vi "Gestion Shielding Box.vi"() -> ()   [LabVIEW 2020]
uses:
  Commun VI/TypeDef/Commande Popup autotest/Commande element autotest.ctl
  <vilib>/Instr/_visa.llb/Select Event Type.ctl
  <vilib>/Instr/_visa.llb/VISA Event Mechanism.ctl
  Action.ctl
  Commande special/Exit.ctl
  IHM/Variable globale.vi
panel:
  out "Element autotest":T1
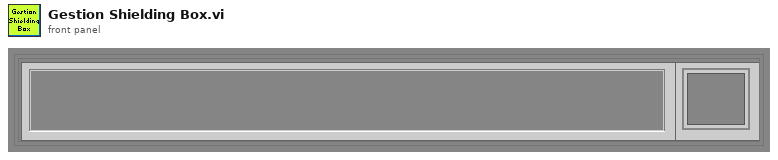
[diagram p1: front panel]
types:
  T1 = typedef "Commande element autotest.ctl" = cluster{"Instrument":string, "Etat":cluster{"Menu déroulant":u16}}
  T2 = typedef "Action.ctl" = enum16{"Open Shielding", "Close Shielding", "Read Status", "Stop Wait Start", "Wait Start", "Wait Close", "Wait Open", "Quit"}
  T3 = typedef "File et notification.ctl" = cluster{"Arret Appli":refnum<notifier>, "Erreur Acqui":refnum<notifier>, "File Event Sequenceur":refnum<queue>, "Liste test à faire":refnum<queue>, "File Event Historique":refnum<queue>, "Variable Global":refnum<notifier>, "Variable stocke retour Etat":refnum<notifier>, "Retour Validation OP":refnum<queue>, "Demande Validation OP":refnum<queue>, "Retour Autotest":refnum<notifier>, "Demande Autotest":refnum<queue>, "Adr Mac Produit":refnum<notifier>, "Autorise commande":refnum<notifier>, "Event Init BLE":refnum<notifier>, "Action Lecture RS":refnum<queue>, "Key produit":refnum<notifier>, "Retour Saisie OP":refnum<queue>, "Demande Saisie OP":refnum<queue>, "Etat flashage":refnum<notifier>, "Code Operateur":refnum<notifier>, "Resultat test Global":refnum<notifier>, "Stop Test":refnum<notifier>, "Init IHM Autotest":refnum<notifier>, "Version test bench":refnum<notifier>, "SN Product":refnum<notifier>, "En erreur":refnum<notifier>, "Affiche Result":refnum<queue>, "S/N PWR":refnum<notifier>, "AppEUI":refnum<notifier>, "Action Lecture Temp":refnum<queue>, "Temp":refnum<notifier>, "AppKey":refnum<notifier>, "OF":refnum<notifier>, "File Commande Shielding":refnum<queue>, "Return Status":refnum<notifier>, "ID Product":refnum<notifier>, "Version FW":refnum<notifier>, "Version HW":refnum<notifier>, "Adresse IHM":refnum<notifier>, "RTC":refnum<notifier>, "S/N Ant":refnum<notifier>, "SN Encode":refnum<notifier>, "Key Product":refnum<notifier>}
  T4 = typedef "Commande Variable Global.ctl" = cluster{"Fichier":cluster{"Chemin Save Historique":path, "Fichier Appplication":string, "Fichier Test":string, "Fichier Langue":string, "Part Number":string, "Fichier Parametre":string, "Chemin Fichier Parametre":path, "Fichier Print":string, "Fichier BDD":string}, "Liaison Serie":cluster{"RS Alimentation":refnum<visa-resource-name>, "RS Multimetre":refnum<k15>, "RS Carte":refnum<visa-resource-name>, "RS Dongle WIFI":refnum<visa-resource-name>, "RS Dongle BLE":refnum<visa-resource-name>, "RSA306":refnum<visa-resource-name>, "RS Printer PCBA":refnum<visa-resource-name>, "RS Golden Sample":refnum<visa-resource-name>, "RS Printer Ass":refnum<visa-resource-name>, "RS Printer Pack":refnum<visa-resource-name>, "RS Sonde Temp":refnum<visa-resource-name>, "RS Multimetre Bis":refnum<k15>, "RS FEASA LED":refnum<visa-resource-name>}, "Liaison DIO":cluster{"Jlink":cluster{"Line":tag, "Nom Voie":string, "Nom device in INI":string}[], "ICD":cluster{"Line":tag, "Nom Voie":string, "Nom device in INI":string}[], "UART":cluster{"Line":tag, "Nom Voie":string, "Nom device in INI":string}[], "Multi1":cluster{"Line":tag, "Nom Voie":string, "Nom device in INI":string}[], "Multi2":cluster{"Line":tag, "Nom Voie":string, "Nom device in INI":string}[], "Multi3":cluster{"Line":tag, "Nom Voie":string, "Nom device in INI":string}[], "DO1":cluster{"Line":tag, "Nom Voie":string, "Nom device in INI":string}[], "DO2":cluster{"Line":tag, "Nom Voie":string, "Nom device in INI":string}[], "DO3":cluster{"Line":tag, "Nom Voie":string, "Nom device in INI":string}[], "AlimProduct":cluster{"Line":tag, "Nom Voie":string, "Nom device in INI":string}[], "SW2":cluster{"Line":tag, "Nom Voie":string, "Nom device in INI":string}[], "SW1":cluster{"Line":tag, "Nom Voie":string, "Nom device in INI":string}[], "Multi220V_CPT":cluster{"Line":tag, "Nom Voie":string, "Nom device in INI":string}[]}, "Variable Programme":T5, "Information Entete":cluster{"Opérateur":string, "Ordre de fabrication":string, "Numéro de lot":string, "Commentaire":string}, "Nom de périphérique DAQmx":tag, "Parameter RF":cluster{"Frequency CW":string, "FrequencyRX":string, "TimeOutRX":string}, "Divers":cluster{"DUT Hub":u32}, "Analogique":cluster{"AI1":cluster{"Voie":tag, "Nom Voie":string, "Nom device in INI":string}[], "Ai2":cluster{"Voie":tag, "Nom Voie":string, "Nom device in INI":string}[], "AI3":cluster{"Voie":tag, "Nom Voie":string, "Nom device in INI":string}[], "AI4":cluster{"Voie":tag, "Nom Voie":string, "Nom device in INI":string}[], "AI5":cluster{"Voie":tag, "Nom Voie":string, "Nom device in INI":string}[], "AI6":cluster{"Voie":tag, "Nom Voie":string, "Nom device in INI":string}[], "AI7":cluster{"Voie":tag, "Nom Voie":string, "Nom device in INI":string}[], "AI8":cluster{"Voie":tag, "Nom Voie":string, "Nom device in INI":string}[], "AO1":cluster{"Voie":tag, "Nom Voie":string, "Nom device in INI":string}[], "AO2":cluster{"Voie":tag, "Nom Voie":string, "Nom device in INI":string}[]}, "Parametre BLE":T8, "Shielding Box":cluster{"Comm":refnum<visa-resource-name>, "Used":bool}, "Challenge Bit":u8[]}
  T5 = typedef "Commande Variables Programme.ctl" = cluster{"Cigarette en cours":i32, "Tableau Resultat test":T6, "Test en cours":i32, "Type test":string, "Type Carte":T7, "Test Select":cluster{"Booléen 4":bool}[]}
  T6 = typedef "Commande tableau Resultat.ctl" = cluster{"Resultat produit":cluster{"Nom test":string, "Result test":bool[], "Nom pointe de test":string[], "Valeur test":string[], "Temps Etape":dbl, "Numero Etape":string[]}[]}[]
  T7 = typedef "Commande Selection produit en cours.ctl" = enum16{"None", "PCBA", "Assembled"}
  T8 = typedef "Comande Variable Globale BLE.ctl" = cluster{"Devices Connect":string[][], "Connection Status":T9, "Handle table":string[][], "Service":string, "characteristic Read":string, "characteristic Write":string, "Port BLE":refnum<visa-resource-name>, "Nb Packet Light":u8}
  T9 = typedef "connection_status_bundle.ctl" = cluster{"MAC Address":string, "cnx handle":u8, "cnx flags":u8, "Address Type":T10, "Connection Interval (ms)":u16, "Timeout(ms)":u16, "Latency":u16, "bonding handle":u8}
  T10 = typedef "address_type.ctl" = u8
  T11 = typedef "Exit.ctl" = bool
  T12 = enum32{"Invalid", "Standard", "Closed", "Hidden", "Minimized", "Maximized"}
  T13 = typedef "VISA Event Mechanism.ctl" = u16
  T14 = typedef "Select Event Type.ctl" = u32
  T15 = typedef "Adresse IHM.ctl" = cluster{"TabGestionScénario":refnum<vi>, "MAJ TabTest":refnum<vi>, "MAJ IHM":refnum<vi>, "BpStop":refnum<vi>, "Autotest OK":refnum<vi>, "BpContinue":refnum<vi>, "BpStart":refnum<vi>, "Action en chinois":refnum<vi>, "Bouton vide":refnum<vi>, "StatusPCB":refnum<vi>, "StatusAssembled":refnum<vi>, "Bouton Exit":refnum<vi>, "Action En cours":refnum<vi>}
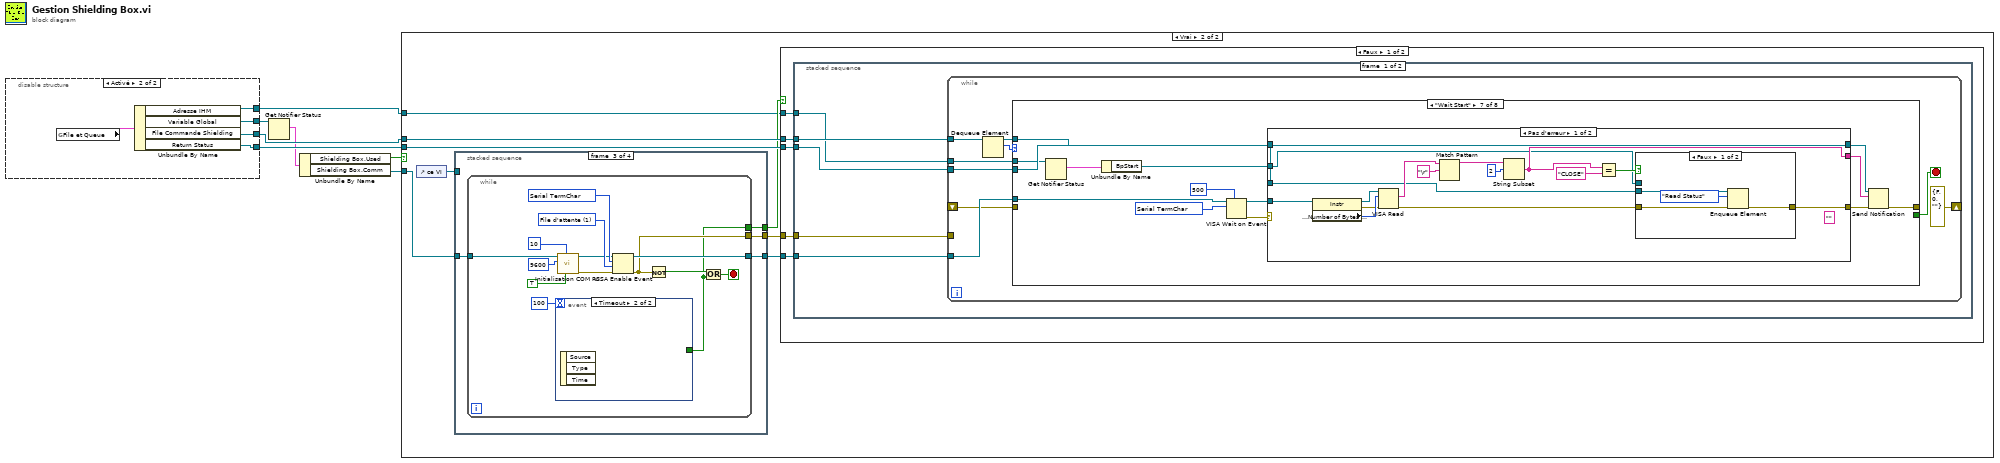
[diagram p0: block diagram]
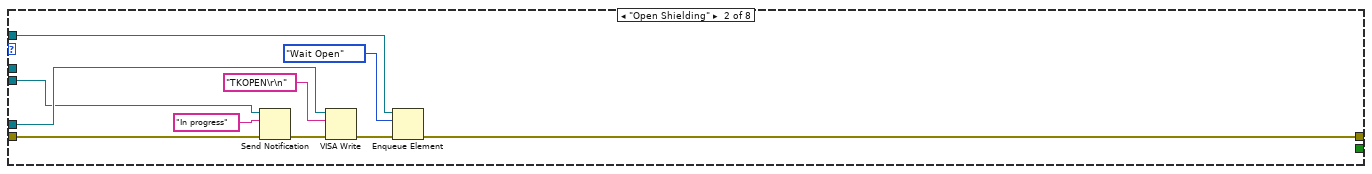
[diagram p4: hidden frame]
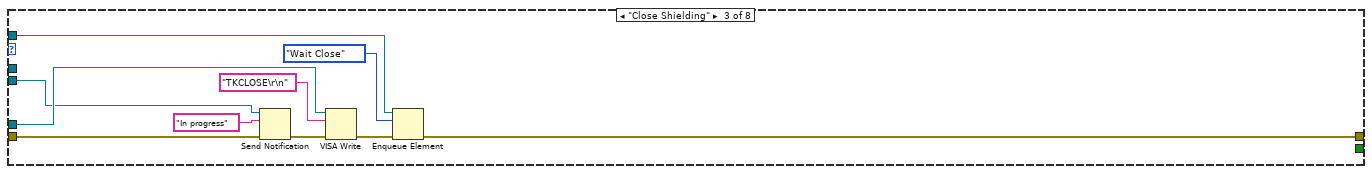
[diagram p5: hidden frame]
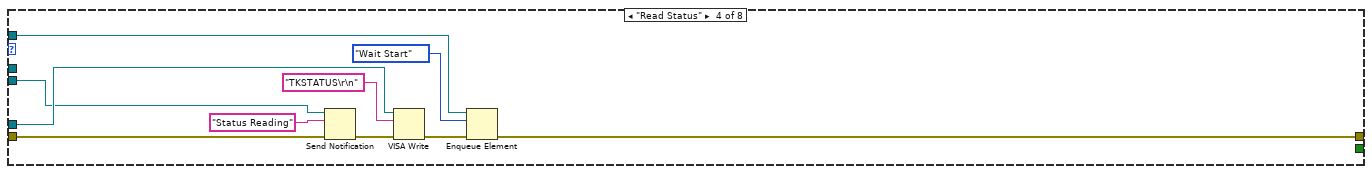
[diagram p6: hidden frame]
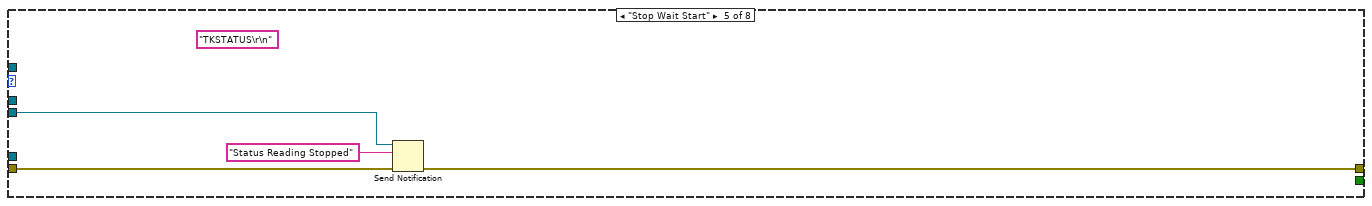
[diagram p7: hidden frame]
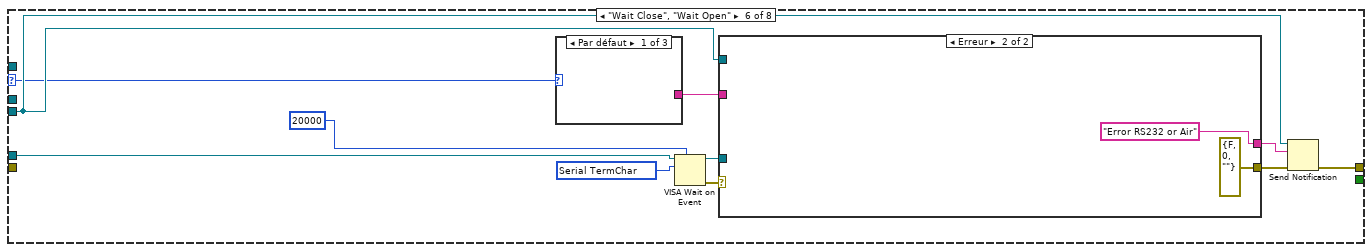
[diagram p8: hidden frame]
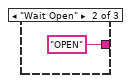
[diagram p9: hidden frame]
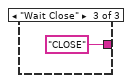
[diagram p10: hidden frame]
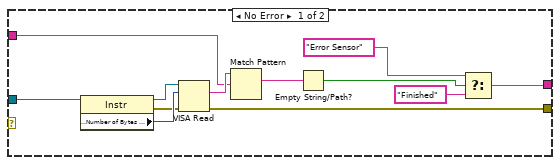
[diagram p11: hidden frame]
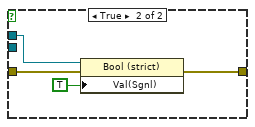
[diagram p12: hidden frame]
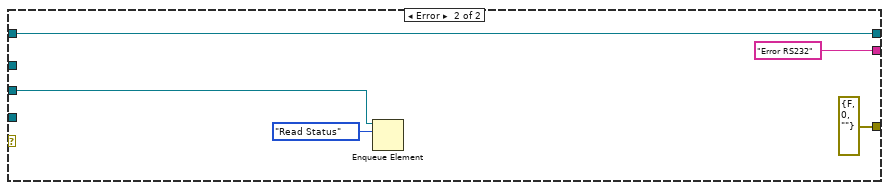
[diagram p13: hidden frame]
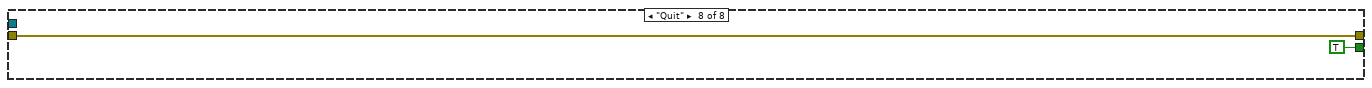
[diagram p14: hidden frame]
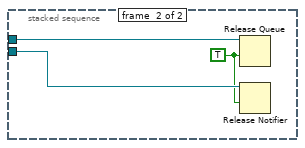
[diagram p15: hidden frame]
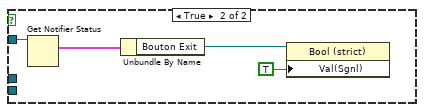
[diagram p16: hidden frame]
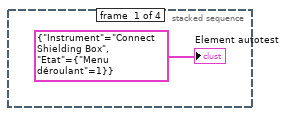
[diagram p17: hidden frame]
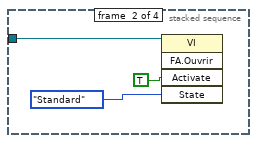
[diagram p18: hidden frame]
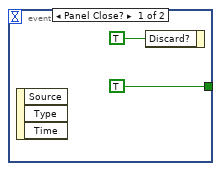
[diagram p19: hidden frame]
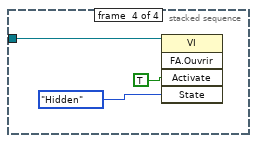
[diagram p20: hidden frame]
diagram:
  n1 = disable-structure shown="Activé" {
    disable-tunnel: [w12 w17] -> w7
    disable-tunnel: [w9 w16] -> w6
    disable-tunnel: [_ w15] -> w5
    disable-tunnel: [_ w14] -> w1
    frame Disabled {
      n2 = Obtain Queue(name (unnamed)="File Commande Shielding" ("nom (aucun)"), element data type=Action."Wait Start") -> (queue out=w12:refnum<queue>)  [unwired: 3 in, 2 out]
      n3 = Obtain Notifier(name (unnamed)="Return Status" ("nom (aucun)"), notification data type="") -> (notifier out=w9:refnum<notifier>)  [unwired: 2 in, 2 out]
    }
    frame Enabled {
      n4 = global read "Variable globale.vi" "File et Queue"() -> (w18:T3)
      n5 = Unbundle By Name(w18) -> ("Adresse IHM"=w14:refnum<notifier>, "Variable Global"=w15:refnum<notifier>, "File Commande Shielding"=w17:refnum<queue>, "Return Status"=w16:refnum<notifier>)
    }
  }
  n6 = Get Notifier Status(notifier=w5) -> (current notification=w3:T4)  [unwired: 1 in, 4 out]
  n7 = Unbundle By Name(w3) -> ("Shielding Box.Used"=w2:bool, "Shielding Box.Comm"=w4:refnum<visa-resource-name>)
  n8 = case shown="Vrai" w2 {
    tunnel: w7 -> [_ w26]
    tunnel: w6 -> [_ w25]
    tunnel: w1 -> [_ w20]
    tunnel: w4 -> [_ w19]
    frame False {
    }
    frame True {
      n9 = control-ref of="ce VI"() -> (w24:refnum<vi>)
      n10 = stacked-sequence {
        tunnel: w24 -> [_ w161 _ w184]
        tunnel: [_ _ w167 _] -> w23
        tunnel: [_ _ w166 _] -> w22
        tunnel: [_ _ w165 _] -> w21
        tunnel: w19 -> [_ _ w164 _]
        frame #0 {
          "Element autotest" <- T1 {"Instrument"="Connect Shielding Box", "Etat"={"Menu déroulant"=1}} ("Element autotest")
        }
        frame #1 {
          n11 = invoke class="VI" method="FA.Ouvrir"(reference=w161, "Activate"=TRUE ("Activer ?"), "State"=T12."Standard" ("État")) -> ()  [unwired: 2 in, 5 out]
        }
        frame #2 {
          n12 = while {
            tunnel: [w172] -> w167
            tunnel: [w174] -> w166
            tunnel: [w170] -> w165
            tunnel: w164 -> [w168]
            stop <- w173 stop-if-true
            w177 = T13 1 items=["File d'attente"=1] ("Mechanism Type")
            w176 = T14 1073684516 items=["Service Request"=1073684491, "Trigger"=3221168138, "Clear"=1073684493, "VXI Signal"=1073684512, "VXI/VME Interrupt"=3221168161, "VXI/VME Sysfail"=1073684509, "VXI/VME Sysreset"=1073684510, "GPIB-CIC"=1073684498, "GPIB-Talk"=1073684499, "GPIB-Listen"=1073684500, "PXI Interrupt"=1073684514, "Serial Break"=1073684515, "Serial TermChar"=1073684516, "Serial CTS"=1073684521, "Serial DSR"=1073684522, "Serial DCD"=1073684524, "Serial RI"=1073684526, "Serial Character"=1073684533, "USB Interrupt"=1073684535, "All Enabled"=1073709055] ("Event Type")
            n13 = event shown="[1] Timeout" {
              selector: _ -> [_ _]
              dyn-events: _ -> [_ _]
              timeout: 100 -> [_ _]
              tunnel: [TRUE _] -> w170
              event Panel Close? {
                n14 = event-data() -> ()  [unwired: 1 in, 3 out]
                n15 = event-data("Discard?"=TRUE ("Rejeter ?")) -> ()  [unwired: 1 in, 1 out]
              }
              event Timeout {
                n16 = event-data() -> ()  [unwired: 1 in, 3 out]
              }
            }
            n17 = call "Initialisation COM RS.vi"("Enable Termination\nChar (T)"=TRUE ("Enable Termination\nChar (T)"), "termination char\n(0xA = '\\n' = LF)"=u8 10 ("termination char\n(0xA = '\\n' = LF)"), "baud rate (9600)"=9600, "Refnum VISA en entrée"=w168) -> ("sortie d'erreur"=w178:errorcluster, "Nom de ressource VISA en sortie"=w175:refnum<visa-resource-name>)  [unwired: 6 in]
            n18 = VISA Enable Event(8:w178, 9:w177, 10:w176, 11:w175) -> (0:w172:errorcluster, 3:w174:refnum<visa-resource-name>)
            n19 = Not(x=w172) -> (.not. x?=w171:bool)
            n20 = Or(x=w171, y=w170) -> (x .or. y?=w173:bool)
          }
        }
        frame #3 {
          n21 = invoke class="VI" method="FA.Ouvrir"(reference=w184, "Activate"=TRUE ("Activer ?"), "State"=T12."Hidden" ("État")) -> ()  [unwired: 2 in, 5 out]
        }
      }
      n22 = case shown="Faux" w21 {
        tunnel: w26 -> [w31 _]
        tunnel: w25 -> [w30 _]
        tunnel: w23 -> [w29 _]
        tunnel: w22 -> [w28 _]
        tunnel: w20 -> [w27 w159]
        frame False {
          n23 = stacked-sequence {
            tunnel: w28 -> [w36 _]
            tunnel: w31 -> [w35 w155]
            tunnel: w29 -> [w34 _]
            tunnel: w30 -> [w33 w154]
            tunnel: w27 -> [w32 _]
            frame #0 {
              n24 = while {
                tunnel: w36 -> [w43]
                tunnel: w35 -> [w45]
                shift-right: [errorcluster {"status"=FALSE, "code"=0, "source"=""} ("error out")] -> _
                shift-left: _ -> [w42]
                tunnel: w34 -> [_]
                tunnel: w33 -> [w39]
                tunnel: w32 -> [w37]
                stop <- w40 stop-if-true
                n25 = Dequeue Element(queue=w45) -> (queue out=w41:refnum<queue>, element=w44:T2)  [unwired: 2 in, 2 out]
                n26 = case shown="\"Wait Start\"" w44 {
                  selector: w44 -> [_ _ _ _ _ w86 _ _]
                  tunnel: w43 -> [_ w56 w66 w76 _ w91 w121 _]
                  tunnel: w42 -> [w46 w54 w58 w68 w78 _ _ w152]
                  tunnel: [w46 w52 w63 w73 w77 w82 w114 w152] -> _
                  tunnel: w41 -> [_ w51 w62 w72 _ _ w110 _]
                  tunnel: [_ _ _ _ _ _ _ TRUE] -> w40
                  tunnel: w39 -> [_ w48 w59 w69 w79 w88 w118 _]
                  tunnel: w37 -> [_ _ _ _ _ _ w115 _]
                  frame Default {
                  }
                  frame "Open Shielding" {
                    n27 = Send Notification(notification="In progress", notifier=w48, error in (no error)=w54) -> (error out=w49:errorcluster)  [unwired: 1 out]
                    n28 = VISA Write(VISA resource name=w56, write buffer="TKOPEN\r\n" ("buffer d'écriture"), error in (no error)=w49) -> (error out=w53:errorcluster)  [unwired: 2 out]
                    n29 = Enqueue Element(queue=w51, element=Action."Wait Open" ("élément"), error in (no error)=w53) -> (error out=w52:errorcluster)  [unwired: 1 in, 2 out]
                  }
                  frame "Close Shielding" {
                    n30 = Send Notification(notification="In progress", notifier=w59, error in (no error)=w58) -> (error out=w57:errorcluster)  [unwired: 1 out]
                    n31 = VISA Write(VISA resource name=w66, write buffer="TKCLOSE\r\n" ("buffer d'écriture"), error in (no error)=w57) -> (error out=w64:errorcluster)  [unwired: 2 out]
                    n32 = Enqueue Element(queue=w62, element=Action."Wait Close" ("élément"), error in (no error)=w64) -> (error out=w63:errorcluster)  [unwired: 1 in, 2 out]
                  }
                  frame "Read Status" {
                    n33 = Send Notification(notification="Status Reading", notifier=w69, error in (no error)=w68) -> (error out=w67:errorcluster)  [unwired: 1 out]
                    n34 = VISA Write(VISA resource name=w76, write buffer="TKSTATUS\r\n" ("buffer d'écriture"), error in (no error)=w67) -> (error out=w74:errorcluster)  [unwired: 2 out]
                    n35 = Enqueue Element(queue=w72, element=Action."Wait Start" ("élément"), error in (no error)=w74) -> (error out=w73:errorcluster)  [unwired: 1 in, 2 out]
                  }
                  frame "Stop Wait Start" {
                    (unwired) "TKSTATUS\r\n" ("buffer d'écriture")
                    n36 = Send Notification(notification="Status Reading Stopped", notifier=w79, error in (no error)=w78) -> (error out=w77:errorcluster)  [unwired: 1 out]
                  }
                  frame "Wait Close", "Wait Open" {
                    w90 = T14 1073684516 items=["Service Request"=1073684491, "Trigger"=3221168138, "Clear"=1073684493, "VXI Signal"=1073684512, "VXI/VME Interrupt"=3221168161, "VXI/VME Sysfail"=1073684509, "VXI/VME Sysreset"=1073684510, "GPIB-CIC"=1073684498, "GPIB-Talk"=1073684499, "GPIB-Listen"=1073684500, "PXI Interrupt"=1073684514, "Serial Break"=1073684515, "Serial TermChar"=1073684516, "Serial CTS"=1073684521, "Serial DSR"=1073684522, "Serial DCD"=1073684524, "Serial RI"=1073684526, "Serial Character"=1073684533, "USB Interrupt"=1073684535, "All Enabled"=1073709055] ("Event Type")
                    n37 = case shown="Par défaut" w86 {
                      tunnel: [_ "OPEN" ("expression régulière") "CLOSE" ("expression régulière")] -> w85
                      frame Default {
                      }
                      frame "Wait Open" {
                      }
                      frame "Wait Close" {
                      }
                    }
                    n38 = VISA Wait on Event(7:u32 20000 ("timeout (0)"), 10:w90, 11:w91) -> (0:w87:errorcluster, 3:w89:refnum<visa-resource-name>)  [unwired: 2 in, 2 out]
                    n39 = case shown="Erreur" w87 {
                      tunnel: w89 -> [w105 _]
                      tunnel: w88 -> [_ _]
                      tunnel: w85 -> [w96 _]
                      tunnel: [w95 "Error RS232 or Air" ("cas faux")] -> w84
                      tunnel: [w94 errorcluster {"status"=FALSE, "code"=0, "source"=""} ("error out")] -> w83
                      frame No Error {
                        n40 = property class="Instr"(reference=w105) -> (reference out=w104:refnum<visa-resource-name>, error out=w101:errorcluster, "Serial Settings:Number of Bytes at Serial Port"=w103:u32)  [unwired: 1 in]
                        n41 = VISA Read(VISA resource name=w104, byte count=w103, error in (no error)=w101) -> (read buffer=w100:string, error out=w94:errorcluster)  [unwired: 2 out]
                        n42 = Match Pattern(string=w100, regular expression=w96) -> (match substring=w102:string)  [unwired: 1 in, 3 out]
                        n43 = Empty String/Path?(string/path=w102) -> (empty?=w97:bool)
                        n44 = Select(t="Error Sensor" ("notification"), s=w97, f="Finished" ("cas faux")) -> (s? t:f=w95:string)
                      }
                      frame Error {
                      }
                    }
                    n45 = Send Notification(notification=w84, notifier=w88, error in (no error)=w83) -> (error out=w82:errorcluster)  [unwired: 1 out]
                  }
                  frame "Wait Start" {
                    w120 = T14 1073684516 items=["Service Request"=1073684491, "Trigger"=3221168138, "Clear"=1073684493, "VXI Signal"=1073684512, "VXI/VME Interrupt"=3221168161, "VXI/VME Sysfail"=1073684509, "VXI/VME Sysreset"=1073684510, "GPIB-CIC"=1073684498, "GPIB-Talk"=1073684499, "GPIB-Listen"=1073684500, "PXI Interrupt"=1073684514, "Serial Break"=1073684515, "Serial TermChar"=1073684516, "Serial CTS"=1073684521, "Serial DSR"=1073684522, "Serial DCD"=1073684524, "Serial RI"=1073684526, "Serial Character"=1073684533, "USB Interrupt"=1073684535, "All Enabled"=1073709055] ("Event Type")
                    n46 = Get Notifier Status(notifier=w115) -> (current notification=w116:T15)  [unwired: 1 in, 4 out]
                    n47 = Unbundle By Name(w116) -> ("BpStart"=w111:refnum<vi>)
                    n48 = VISA Wait on Event(7:u32 500 ("timeout (0)"), 10:w120, 11:w121) -> (0:w117:errorcluster, 3:w119:refnum<visa-resource-name>)  [unwired: 2 in, 2 out]
                    n49 = case shown="Pas d'erreur" w117 {
                      tunnel: w119 -> [w137 _]
                      tunnel: w118 -> [w128 w148]
                      tunnel: [w127 "Error RS232" ("cas faux")] -> w112
                      tunnel: [w122 errorcluster {"status"=FALSE, "code"=0, "source"=""} ("error out")] -> w109
                      tunnel: [w128 w148] -> w113
                      tunnel: w111 -> [w125 _]
                      tunnel: w110 -> [w123 w146]
                      frame No Error {
                        (unwired) "" ("sous-chaîne")
                        n50 = property class="Instr"(reference=w137) -> (reference out=w136:refnum<visa-resource-name>, error out=w134:errorcluster, "Serial Settings:Number of Bytes at Serial Port"=w135:u32)  [unwired: 1 in]
                        n51 = VISA Read(VISA resource name=w136, byte count=w135, error in (no error)=w134) -> (read buffer=w133:string, error out=w124:errorcluster)  [unwired: 2 out]
                        n52 = Match Pattern(string=w133, regular expression="\r" ("expression régulière")) -> (before substring=w131:string)  [unwired: 1 in, 3 out]
                        n53 = String Subset(string=w131, offset (0)=2) -> (substring=w127:string)  [unwired: 1 in]
                        n54 = Equal?(x=w127, y="CLOSE") -> (x = y?=w126:bool)
                        n55 = case shown="Faux" w126 {
                          tunnel: w125 -> [_ w145]
                          tunnel: w124 -> [w141 w143]
                          tunnel: [w140 w142] -> w122
                          tunnel: w123 -> [w139 _]
                          frame False {
                            n56 = Enqueue Element(queue=w139, element=Action."Read Status" ("élément"), error in (no error)=w141) -> (error out=w140:errorcluster)  [unwired: 1 in, 2 out]
                          }
                          frame True {
                            n57 = property class="Bool (strict)"(reference=w145, error in=w143, "Val(Sgnl)"=T11 TRUE ("Valeur (Signalisation)")) -> (error out=w142:errorcluster)  [unwired: 1 out]
                          }
                        }
                      }
                      frame Error {
                        n58 = Enqueue Element(queue=w146, element=Action."Read Status" ("élément")) -> ()  [unwired: 2 in, 3 out]
                      }
                    }
                    n59 = Send Notification(notification=w112, notifier=w113, error in (no error)=w109) -> (error out=w114:errorcluster)  [unwired: 1 out]
                  }
                  frame "Quit" {
                  }
                }
              }
            }
            frame #1 {
              w153 = TRUE ("forcer la destruction ? (F)")
              n60 = Release Queue(queue=w155, force destroy? (F)=w153) -> ()  [unwired: 1 in, 3 out]
              n61 = Release Notifier(notifier=w154, force destroy? (F)=w153) -> ()  [unwired: 1 in, 3 out]
            }
          }
        }
        frame True {
          n62 = Get Notifier Status(notifier=w159) -> (current notification=w156:T15)  [unwired: 1 in, 4 out]
          n63 = Unbundle By Name(w156) -> ("Bouton Exit"=w158:refnum<vi>)
          n64 = property class="Bool (strict)"(reference=w158, "Val(Sgnl)"=T11 TRUE ("Valeur (Signalisation)")) -> ()  [unwired: 1 in, 2 out]
        }
      }
    }
  }
